vi "HEWH Sum Total Gallons.vi"(8 "error in (no error)":errorcluster, 11 "Water Draw Amounts-(Gal)":dbl[](array[numeric])) -> (0 "error out":errorcluster, 3 "Total Gallons":dbl)   [LabVIEW 2023]
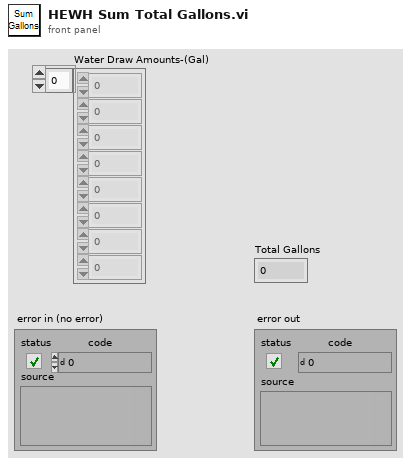
[diagram p1: front panel]
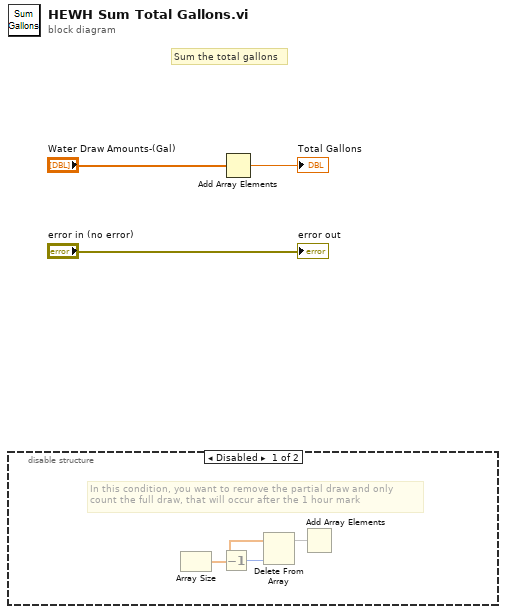
[diagram p0: block diagram]
diagram:
  # "Sum the total gallons"
  n1 = disable-structure shown="Disabled" {
    frame Disabled {
      # "In this condition, you want to remove the partial draw and only\ncount the full draw, that will occur after the 1 hour mark"
      n2 = Array Size() -> (array=w7:dbl[], size(s)=w4:i32)
      n3 = Decrement(x=w4) -> (x-1=w5:i32)
      n4 = Delete From Array(array=w7, index=w5) -> (array with subset deleted=w6)  [unwired: 1 in, 1 out]
      n5 = Add Array Elements(numeric array=w6) -> (sum=w8:dbl)
    }
    frame Enabled {
    }
  }
  n6 = Add Array Elements(numeric array="Water Draw Amounts-(Gal)") -> (sum=→"Total Gallons":dbl)
  "error out" <- "error in (no error)"
